vi "PH_ImageCoG_Plotter.PC set selected Cam.vi"(0 "VI in":refnum<vi>, 2 "Camera to select":string, 5 "error in (no error)":errorcluster) -> (14 "VI out":refnum<vi>, 19 "error out":errorcluster)   [LabVIEW 2014, in "PH_ImageCoG_Plotter.lvlib"]
uses:
  PH_ImageCoG_Plotter.lvlib
  PH_Basics/PH_Common/DIM/PH_DIM.Event Declarer.ctl
  CS_Core/BaseProcess/BaseProcess.lvlib
  PH_Basics/PH_Common/PH_Common.lvlib
  PH_Basics/PH_Img_BaseClass/PH_Img_BaseClass.lvlib
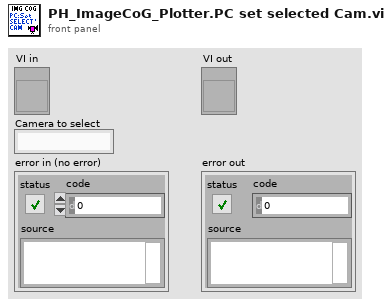
[diagram p1: front panel]
types:
  T1 = typedef "PH_Common.lvlib/PH_DIM.Event Declarer.ctl" = cluster{"Service Name":string, "Selector":string}
  T2 = typedef "PH_Img_BaseClass.lvlib/PH_Img_BaseClass.i attribute.ctl" = cluster{"GUI Refs":T3, "Timeout Image [ms]":i32, "Default Periodic Period [ms]":i32, "Camera":cluster{"Instancename":string, "Notifier":refnum<notifier>}, "Palette":T4, "Cam Settings":cluster{"Cam ID":string, "Gain":dbl, "Brightness":dbl, "Shutter":dbl, "Cam Info Failure":bool, "Mode":i32}}
  T3 = typedef "PH_Img_BaseClass.lvlib/PH_Img_BaseClass.GUI Refs.ctl" = cluster{"Timeout":refnum<vi>, "Image":refnum<vi>, "Palette":refnum<vi>, "Timeout Set":refnum<vi>}
  T4 = typedef "PH_Img_BaseClass.lvlib/PH_Img_BaseClass.Palette.ctl" = i32
  T5 = typedef "PH_ImageCoG_Plotter.lvlib/PH_ImageCoG_Plotter.i attribute.ctl" = cluster{"GUI Refs":cluster{"Delete":refnum<vi>, "Calibration status":refnum<vi>, "BI subtracted":refnum<vi>, "calc Beam Anal":refnum<vi>, "CoG - x":refnum<vi>, "CoG - y":refnum<vi>, "Type":refnum<vi>, "Center":refnum<vi>, "exp - X":refnum<vi>, "exp - Y":refnum<vi>, "Delta - X":refnum<vi>, "Delta - Y":refnum<vi>, "Available Cams":refnum<vi>, "CoG X":refnum<vi>, "CoG Y":refnum<vi>, "Delta X":refnum<vi>, "Delta Y":refnum<vi>, "Export Data":refnum<vi>, "Calibration data":refnum<vi>}, "Calibration":cluster{"Status":T6, "Calibration data":T7, "Calibration Data File":path}, "Beam Analysis":cluster{"on":bool, "exp - X":i32, "exp - Y":i32, "Type":bool, "Data":cluster{"current time":timestamp, "CoG-x":dbl, "CoG-y":dbl, "Delta-x":dbl, "Delta-y":dbl}[], "Datasets strored":i32, "Dataarray Size":i32}, "Cam instances":string[], "DIM Service Events":T8[], "Images":cluster{"Background":T11, "OP":T11, "GUI":T11}}
  T6 = typedef "PH_StatusHandler.lvlib/PH_StatusHandler.Status.ctl" = i16
  T7 = typedef "PH_ImageCalibrator.lvlib/PH_ImageCalibrator.Calibration Data.ctl" = cluster{"Date":string, "Time":string, "Cam Settings":cluster{"Cam ID":string, "Gain":dbl, "Brightness":dbl, "Shutter":dbl, "Cam Error":bool, "Mode":i32}, "Background Image":cluster{"Image":dbl[][], "Image Error":bool}, "Linear Calibration":cluster{"Calibration Factor":dbl, "not mm or mrad":bool}, "Energy Calibration":cluster{"Calibration Factor":dbl, "no mJ":bool}}
  T8 = typedef "BaseProcess.lvlib/BaseProcess.event definition.ctl" = cluster{"CAEEvtDef":T9, "Data Descriptor":T10}
  T9 = typedef "CAEObj.lvlib/CAEObj.event definition.ctl" = cluster{"URL":string, "enable":bool, "ignoreResID":bool}
  T10 = typedef "BaseProcess.lvlib/BaseProcess.descriptor string definition.ctl" = string
  T11 = typedef "IMAQ Image.ctl" = refnum<image>
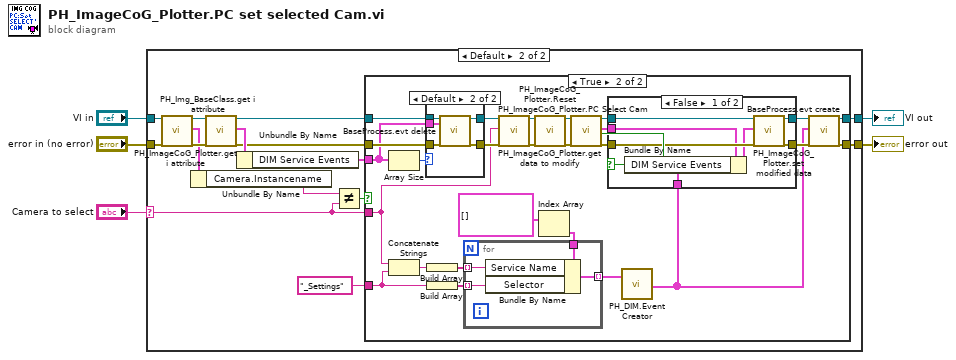
[diagram p0: block diagram]
diagram:
  n1 = case shown="Default" "Camera to select" {
    selector: "Camera to select" -> [_ w16]
    tunnel: "error in (no error)" -> [w6 w20]
    tunnel: "VI in" -> [w7 w11]
    tunnel: [w7 w22] -> w3
    tunnel: [w6 w21] -> w4
    frame "", "N/A" {
    }
    frame Default {
      n2 = call "PH_Img_BaseClass.get i attribute.vi"("i ref in"=w11, "error in (no error)"=w20) -> ("i ref out"=w10:refnum<vi>, "i attribute"=w9:T2, "error out"=w12:errorcluster)  [unwired: 15 in]
      n3 = Unbundle By Name(w9) -> ("Camera.Instancename"=w8:string)
      n4 = call "PH_ImageCoG_Plotter.get i attribute.vi"("i ref in"=w10, "error in (no error)"=w12) -> ("i ref out"=w17:refnum<vi>, "i attribute"=w19:T5, "error out"=w18:errorcluster)  [unwired: 15 in]
      n5 = Unbundle By Name(w19) -> ("DIM Service Events"=w14:T8[])
      n6 = Not Equal?(x=w8, y=w16) -> (x != y?=w15:bool)
      n7 = case shown="True" w15 {
        tunnel: [w24 w49] -> w22
        tunnel: [w23 w48] -> w21
        tunnel: w18 -> [w23 w47]
        tunnel: w17 -> [w24 w45]
        tunnel: w16 -> [_ w25]
        tunnel: w14 -> [_ w38]
        tunnel: "_Settings" ("string") -> [_ w37]
        frame False {
        }
        frame True {
          n8 = Array Size(array=w38) -> (size(s)=w39:i32)
          n9 = Concatenate Strings(w25, w37) -> (w43:string)
          n10 = case shown="Default" w39 {
            tunnel: w47 -> [w61 w67]
            tunnel: [w61 w66] -> w46
            tunnel: w45 -> [w62 w65]
            tunnel: [w62 w64] -> w44
            tunnel: w38 -> [_ w63]
            frame 0 {
            }
            frame Default {
              n11 = call "BaseProcess.evt delete.vi"("i ref in"=w65, "events"=w63, "error in (no error)"=w67) -> ("i ref out"=w64:refnum<vi>, "error out"=w66:errorcluster)  [unwired: 13 in, 2 out]
            }
          }
          n12 = Build Array(w43) -> (w41:string[])
          n13 = Build Array(w37) -> (w40:string[])
          n14 = call "PH_ImageCoG_Plotter.PC Select Cam.vi"("i ref in"=w44, "Cam Instance"=w25, "error in (no error)"=w46) -> ("i ref out"=w50:refnum<vi>, "error out"=w51:errorcluster)  [unwired: 15 in]
          n15 = call "PH_ImageCoG_Plotter.Reset.vi"("i ref in"=w50, "error in"=w51) -> ("i ref out"=w34:refnum<vi>, "error out"=w32:errorcluster)  [unwired: 16 in]
          n16 = Index Array(array=T1[] [] ("Services")) -> (element=w26:T1)  [unwired: 1 in]
          n17 = for {
            tunnel: w26 -> [w71]
            tunnel: [w70] -> w42 mode=indexing
            tunnel: w41 -> [w69] mode=indexing
            tunnel: w40 -> [w68] mode=indexing
            n18 = Bundle By Name(cluster=w71, "Service Name"=w69, "Selector"=w68) -> (w70:T1)
          }
          n19 = call "PH_ImageCoG_Plotter.get data to modify.vi"("i ref in"=w34, "error in (no error)"=w32) -> ("i ref out"=w35:refnum<vi>, "i attribute"=w29:T5, "timed out"=w30:bool, "error out"=w36:errorcluster)  [unwired: 14 in]
          n20 = call "PH_DIM.Event Creator.vi"("Trendmessage Services"=w42) -> ("DIM Service Events"=w28:T8[])  [unwired: 18 in]
          n21 = case shown="False" w30 {
            tunnel: w36 -> [w58 w59]
            tunnel: w35 -> [w57 w60]
            tunnel: [w56 w60] -> w33
            tunnel: [w55 w59] -> w31
            tunnel: w29 -> [w54 _]
            tunnel: w28 -> [w52 _]
            frame False {
              n22 = Bundle By Name(cluster=w54, "DIM Service Events"=w52) -> (w53:T5)
              n23 = call "PH_ImageCoG_Plotter.set modified data.vi"("i ref in"=w57, "i attribute"=w53, "error in (no error)"=w58) -> ("i ref out"=w56:refnum<vi>, "error out"=w55:errorcluster)  [unwired: 15 in]
            }
            frame True {
            }
          }
          n24 = call "BaseProcess.evt create.vi"("i ref in"=w33, "newEvents"=w28, "error in (no error)"=w31) -> ("i ref out"=w49:refnum<vi>, "error out"=w48:errorcluster)  [unwired: 13 in, 2 out]
        }
      }
    }
  }
  "error out" <- w4
  "VI out" <- w3
